vi "_checkW&R_EEPROM_vna_wmg - 副本.vi"(3 "EEPROMCheck":string[][](array[string])=[["1", "0", "3"], ["1", "10", "14"], ["3", "2", "4"]], 4 "readout":string[][](array[string])=[["1", "1", "2"], ["1", "1", "2"], ["1", "1", "2"], ["1", "1", "2"], ["1", "1", "2"], ["1", "1", "2"], ["1", "1", "2"], ["1", "1", "2"], ["1", "1", "2"], ["1", "1", "2"], ["1", "1", "2"], ["1", "1", "2"], ["1", "1", "2"], ["1", "1", "2"], ["1", "1", "2"], ["1", "1", "2"]], 5 "info_write":string[][](array[string])=[["3", "1", "2"], ["3", "1", "2"], ["3", "1", "5"], ["3", "1", "5"], ["1", "1", "5"], ["1", "1", "2"], ["1", "1", "2"], ["1", "1", "2"], ["1", "1", "2"], ["1", "1", "2"], ["3", "1", "2"], ["3", "1", "2"], ["3", "1", "2"], ["3", "1", "2"], ["3", "1", "2"], ["1", "1", "2"]]) -> (0 "message":string, 1 "result_A":bool[](array[boolean]), 2 "result":bool)   [LabVIEW 2011]
panel:
  out "message_1":string
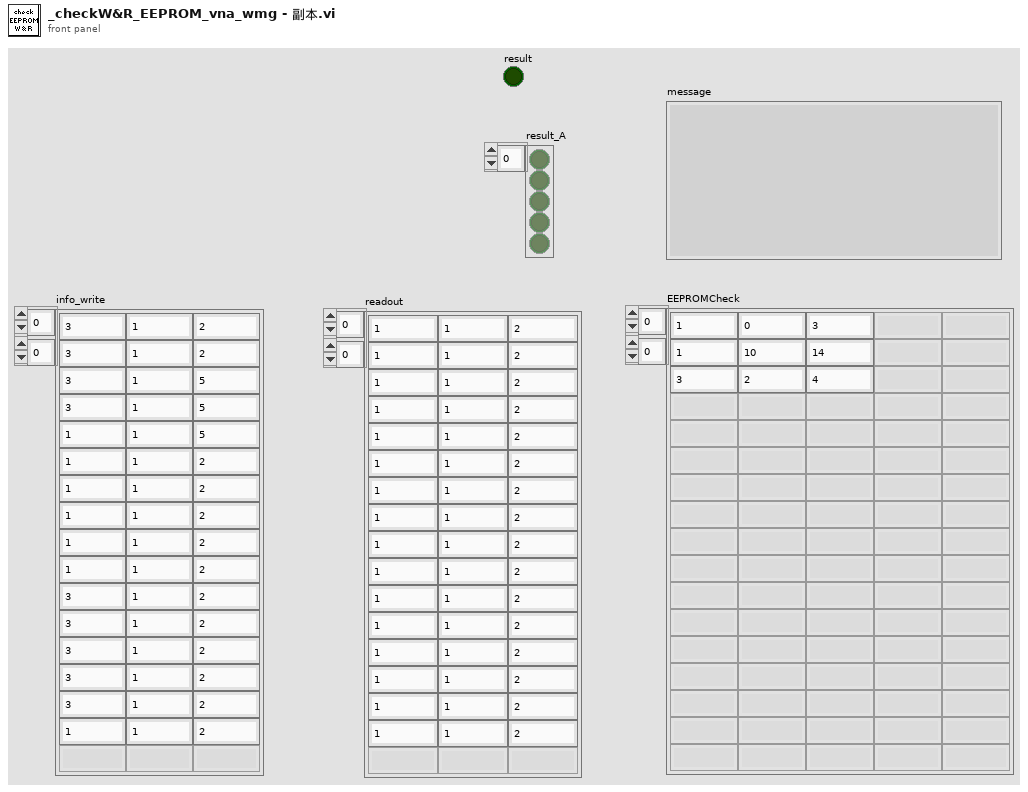
[diagram p1: front panel]
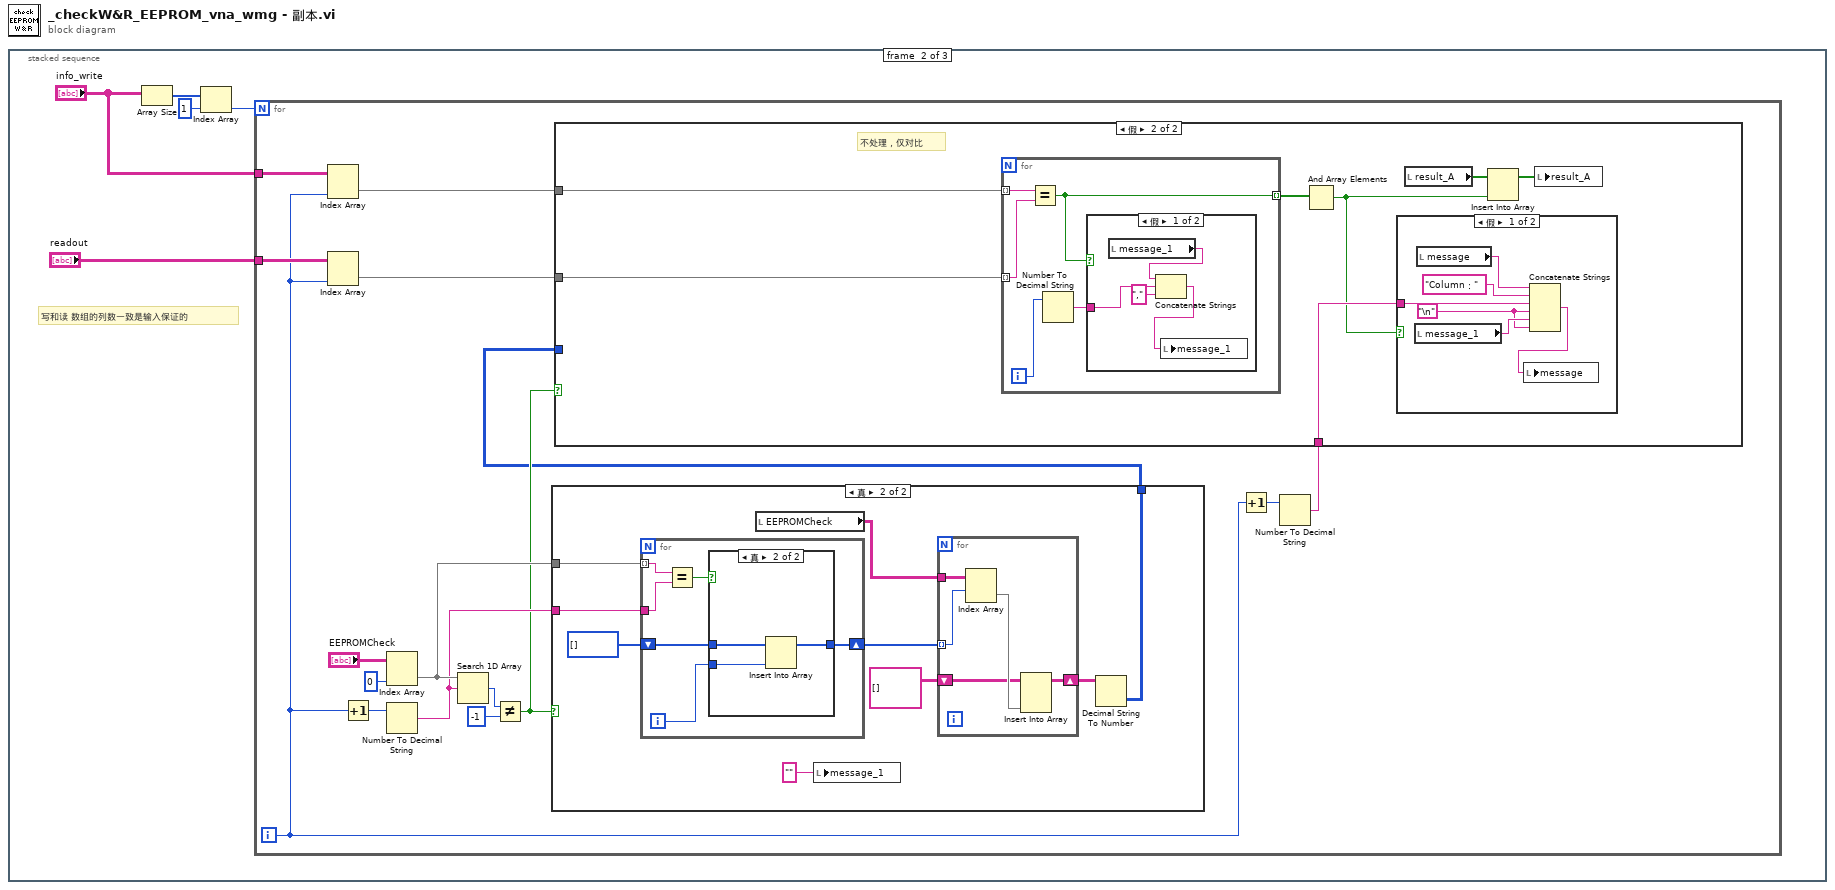
[diagram p0: block diagram]
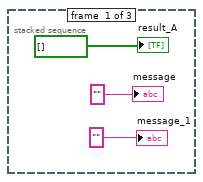
[diagram p2: hidden frame]
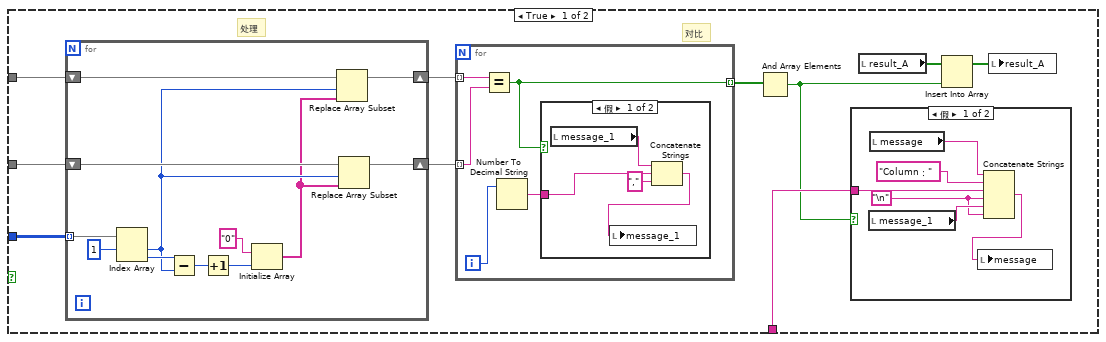
[diagram p3: hidden frame]
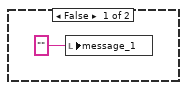
[diagram p8: hidden frame]
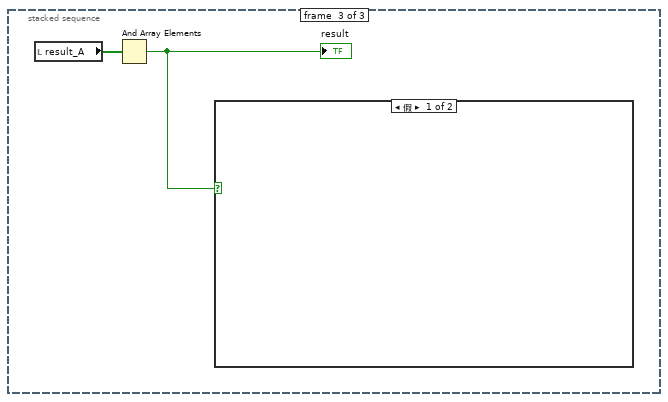
[diagram p10: hidden frame]
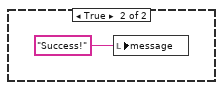
[diagram p11: hidden frame]
diagram:
  n1 = stacked-sequence {
    frame #0 {
      "result_A" <- bool[] []
      "message" <- ""
      "message_1" <- "" ("message_1")
    }
    frame #1 {
      # "写和读 数组的列数一致是输入保证的"
      n2 = Array Size(array="info_write") -> (size(s)=w8:i32[])
      n3 = Index Array(array=w8, index=1 ("索引")) -> (element=w6:i32)
      n4 = for {
        N: w6 -> [_]
        tunnel: "info_write" -> [w24]
        tunnel: "readout" -> [w23]
        i -> [w11]
        n5 = Index Array(array=w24, index (col)=w11) -> (element=w13:string[])  [unwired: 1 in]
        n6 = Index Array(array=w23, index (col)=w11) -> (element=w12:string[])  [unwired: 1 in]
        n7 = Increment(x=w11) -> (x+1=w20:i32)
        n8 = Index Array(array="EEPROMCheck", index (col)=0 ("禁用的索引 (列)")) -> (element=w17:string[])  [unwired: 1 in]
        n9 = Number To Decimal String(number=w20) -> (decimal integer string=w16:string)  [unwired: 1 in]
        n10 = Search 1D Array(1D array=w17, element=w16) -> (index of element=w19:i32)  [unwired: 1 in]
        n11 = Not Equal?(x=w19, y=-1) -> (x != y?=w15:bool)
        n12 = case shown="真" w15 {
          tunnel: w17 -> [_ w93]
          tunnel: w16 -> [_ w92]
          tunnel: [_ w86] -> w14
          frame False {
            n13 = local write "message_1"("") -> ()
          }
          frame True {
            n14 = for {
              tunnel: w93 -> [w104] mode=indexing
              tunnel: w92 -> [w103]
              shift-right: [w100] -> w90
              shift-left: i32[] [] -> [w101]
              i -> [w99]
              n15 = Equal?(x=w104, y=w103) -> (x = y?=w102:bool)
              n16 = case shown="真" w102 {
                tunnel: w101 -> [w105 w108]
                tunnel: [w105 w107] -> w100
                tunnel: w99 -> [_ w106]
                frame False {
                }
                frame True {
                  n17 = Insert Into Array(array=w108, new element=w106) -> (w107:i32[])  [unwired: 1 in]
                }
              }
            }
            n18 = local read "EEPROMCheck"() -> (w89:string[][])
            n19 = local write "message_1"("") -> ()
            n20 = for {
              tunnel: w90 -> [w97] mode=indexing
              tunnel: w89 -> [w98]
              shift-right: [w94] -> w87
              shift-left: string[][] [] ("EEPROMCheck 2") -> [w95]
              n21 = Index Array(array=w98, index (row)=w97) -> (element=w96:string[])  [unwired: 1 in]
              n22 = Insert Into Array(array=w95, new element=w96) -> (w94:string[][])  [unwired: 2 in]
            }
            n23 = Decimal String To Number(string=w87) -> (number=w86:i32[][])  [unwired: 2 in, 1 out]
          }
        }
        n24 = Increment(x=w11) -> (x+1=w9:i32)
        n25 = Number To Decimal String(number=w9) -> (decimal integer string=w10:string)  [unwired: 1 in]
        n26 = case shown="假" w15 {
          tunnel: w14 -> [w34 _]
          tunnel: w13 -> [w33 w63]
          tunnel: w12 -> [w32 w62]
          tunnel: w10 -> [w28 w67]
          frame True {
            # "处理"
            # "对比"
            n27 = for {
              tunnel: w34 -> [w61] mode=indexing
              shift-right: [w51] -> w31
              shift-left: w33 -> [w59]
              shift-right: [w50] -> w30
              shift-left: w32 -> [w54]
              n28 = Index Array(array=w61, index #1=1 ("索引")) -> (element #1=w53:i32, element #2=w58:i32)  [unwired: 1 in]
              n29 = Subtract(x=w58, y=w53) -> (x-y=w57:i32)
              n30 = Increment(x=w57) -> (x+1=w56:i32)
              n31 = Initialize Array("0", w56) -> (w52:string[])
              n32 = Replace Array Subset(array=w59, new element=w52, index=w53) -> (w51:string[])
              n33 = Replace Array Subset(array=w54, new element=w52, index=w53) -> (w50:string[])
            }
            n34 = for {
              tunnel: w31 -> [w45] mode=indexing
              tunnel: w30 -> [w44] mode=indexing
              tunnel: [w43] -> w29 mode=indexing
              i -> [w42]
              n35 = Equal?(x=w45, y=w44) -> (x = y?=w43:bool)
              n36 = Number To Decimal String(number=w42) -> (decimal integer string=w41:string)  [unwired: 1 in]
              n37 = case shown="假" w43 {
                tunnel: w41 -> [w48 _]
                frame False {
                  n38 = local read "message_1"() -> (w49:string)
                  n39 = Concatenate Strings(w49, w48, "," ("字符串")) -> (w46:string)
                  n40 = local write "message_1"(w46) -> ()
                }
                frame True {
                }
              }
            }
            n41 = And Array Elements(Boolean array=w29) -> (logical AND=w26:bool)
            n42 = case shown="假" w26 {
              tunnel: w28 -> [w40 _]
              frame False {
                w38 = "\n"
                n43 = local read "message_1"() -> (w39:string)
                n44 = local read "message"() -> (w35:string)
                n45 = Concatenate Strings(w35, "Column：", w40, w38, w39, w38) -> (w37:string)
                n46 = local write "message"(w37) -> ()
              }
              frame True {
              }
            }
            n47 = local read "result_A"() -> (w27:bool[])
            n48 = Insert Into Array(array=w27, new element=w26) -> (w25:bool[])  [unwired: 1 in]
            n49 = local write "result_A"(w25) -> ()
          }
          frame False {
            # "不处理，仅对比"
            n50 = for {
              tunnel: w63 -> [w79] mode=indexing
              tunnel: w62 -> [w78] mode=indexing
              tunnel: [w77] -> w68 mode=indexing
              i -> [w76]
              n51 = Equal?(x=w79, y=w78) -> (x = y?=w77:bool)
              n52 = Number To Decimal String(number=w76) -> (decimal integer string=w75:string)  [unwired: 1 in]
              n53 = case shown="假" w77 {
                tunnel: w75 -> [w83 _]
                frame False {
                  n54 = local read "message_1"() -> (w80:string)
                  n55 = Concatenate Strings(w80, w83, "," ("字符串")) -> (w81:string)
                  n56 = local write "message_1"(w81) -> ()
                }
                frame True {
                }
              }
            }
            n57 = And Array Elements(Boolean array=w68) -> (logical AND=w65:bool)
            n58 = case shown="假" w65 {
              tunnel: w67 -> [w73 _]
              frame False {
                w71 = "\n"
                n59 = local read "message_1"() -> (w72:string)
                n60 = local read "message"() -> (w69:string)
                n61 = Concatenate Strings(w69, "Column：", w73, w71, w72, w71) -> (w70:string)
                n62 = local write "message"(w70) -> ()
              }
              frame True {
              }
            }
            n63 = local read "result_A"() -> (w66:bool[])
            n64 = Insert Into Array(array=w66, new element=w65) -> (w64:bool[])  [unwired: 1 in]
            n65 = local write "result_A"(w64) -> ()
          }
        }
      }
    }
    frame #2 {
      n66 = local read "result_A"() -> (w110:bool[])
      n67 = And Array Elements(Boolean array=w110) -> (logical AND=w109:bool)
      "result" <- w109
      n68 = case shown="假" w109 {
        frame False {
        }
        frame True {
          n69 = local write "message"("Success!" ("message")) -> ()
        }
      }
    }
  }
